vi "Read Voltage From Channel.vi"(8 "error in (no error)":errorcluster, 10 "Channel":u8, 11 "IRead Voltage Multichannel in":refnum<class "Scope Base.lvclass">) -> (0 "error out":errorcluster, 2 "Voltage":dbl format="%#_g V", 3 "IRead Voltage Multichannel out":refnum<class "Scope Base.lvclass">)   [LabVIEW 2023, in "Scope.lvlib" / "Scope Base.lvlib" / "Scope Base.lvclass"]
uses:
  Scope Base.lvclass
  Interfaces/IConfigure MultiChannel Voltmeter/IConfigure MultiChannel Voltmeter.lvclass
  Scope Base.lvclass/Scope Base.ctl
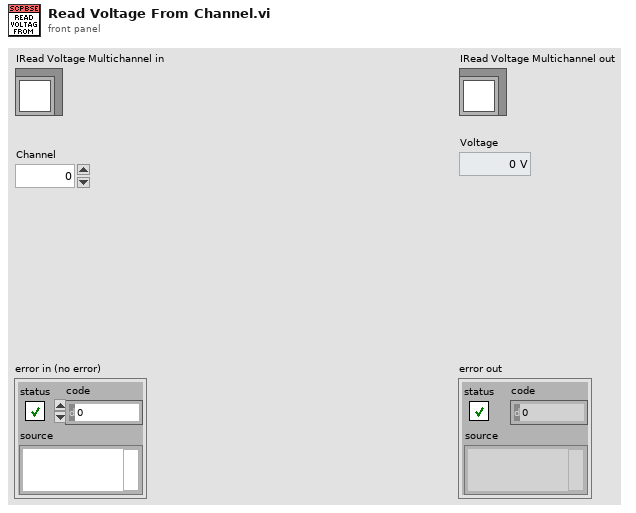
[diagram p1: front panel]
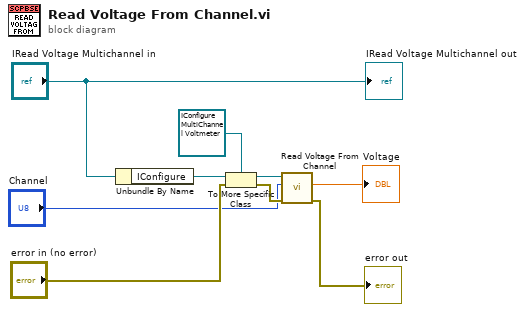
[diagram p0: block diagram]
diagram:
  n1 = Unbundle By Name("IRead Voltage Multichannel in") -> ("IConfigure"=w6:refnum<class "IConfigure.lvclass">)
  n2 = To More Specific Class(target class=refnum<class "IConfigure MultiChannel Voltmeter.lvclass"> refnum ("IConfigure Voltmeter.lvclass"), reference=w6, error in="error in (no error)") -> (specific class reference=w8:refnum<class "IConfigure MultiChannel Voltmeter.lvclass">, error out=w7:errorcluster)
  n3 = call-dynamic "Read Voltage From Channel.vi"("error in (no error)"=w7, "Numeric"="Channel", "IConfigure MultiChannel Voltmeter in"=w8) -> ("error out"=→"error out":errorcluster, "Voltage"=→"Voltage":dbl)  [unwired: 6 in, 1 out]
  "IRead Voltage Multichannel out" <- "IRead Voltage Multichannel in"
